vi "CRYPIC CLOSE SPLITER.vi"(10 "tSpliter":T1) -> (2 "tSpliter_Out":T1)   [LabVIEW 2013]
uses:
  CRYMain Sub Window Global.vi
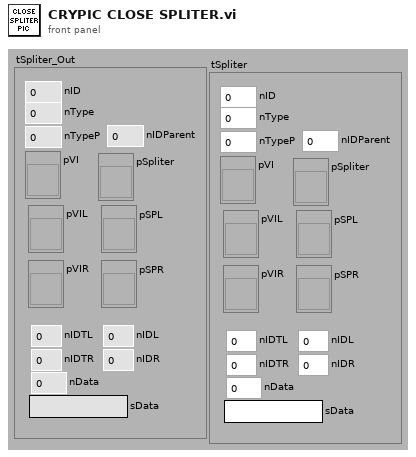
[diagram p1: front panel]
types:
  T1 = cluster{"nType":i32, "nTypeP":i32, "pVI":refnum<vi>, "pSpliter":refnum<vi>, "pSPL":refnum<vi>, "pVIL":refnum<vi>, "pSPR":refnum<vi>, "pVIR":refnum<vi>, "nIDTL":i32, "nIDL":i32, "nIDTR":i32, "nIDR":i32, "nID":i32, "nIDParent":i32, "nData":i32, "sData":string}
  T2 = cluster{"nID":i32[], "Spliter":cluster{"nType":i32, "nTypeP":i32, "pVI":refnum<vi>, "pSpliter":refnum<vi>, "pSPL":refnum<vi>, "pVIL":refnum<vi>, "pSPR":refnum<vi>, "pVIR":refnum<vi>, "nIDTL":i32, "nIDL":i32, "nIDTR":i32, "nIDR":i32, "nID":i32, "nIDParent":i32, "nData":i32, "sData":string}[]}
  T3 = cluster{"nType":i32, "nTypeP":i32, "pVI":refnum<vi>, "pSpliter":refnum<vi>, "pSPL":refnum<vi>, "pVIL":refnum<vi>, "pSPR":refnum<vi>, "pVIR":refnum<vi>, "nIDTL":i32, "nIDL":i32, "nIDTR":i32, "nIDR":i32, "nID":i32, "nIDParent":i32, "nData":i32, "sData":string}[]
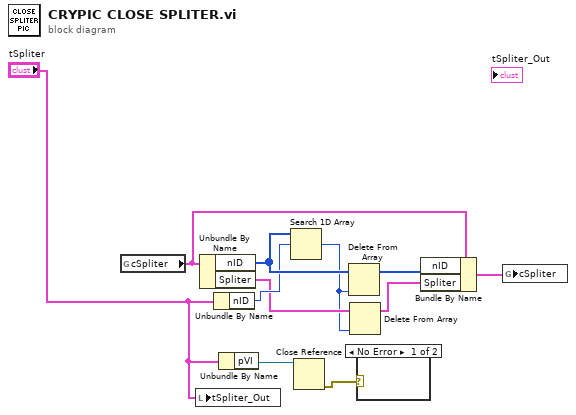
[diagram p0: block diagram]
diagram:
  n1 = global read "CRYMain Sub Window Global.vi" "cSpliter"() -> (w10:T2)
  n2 = local write "tSpliter_Out"("tSpliter") -> ()
  n3 = Unbundle By Name(w10) -> ("nID"=w9:i32[], "Spliter"=w6:T3)
  n4 = Unbundle By Name("tSpliter") -> ("nID"=w8:i32)
  n5 = Unbundle By Name("tSpliter") -> ("pVI"=w2:refnum<vi>)
  n6 = Search 1D Array(1D array=w9, element=w8) -> (index of element=w5:i32)  [unwired: 1 out]
  n7 = Close Reference(reference=w2) -> (error out=w1:errorcluster)  [unwired: 1 in]
  n8 = Delete From Array(array=w9, index=w5) -> (array with subset deleted=w11:i32[])  [unwired: 1 in, 1 out]
  n9 = Delete From Array(array=w6, index=w5) -> (array with subset deleted=w7:T3)  [unwired: 1 in, 1 out]
  n10 = case shown="No Error" w1 {
    frame No Error {
    }
    frame Error {
    }
  }
  n11 = Bundle By Name(cluster=w10, "nID"=w11, "Spliter"=w7) -> (w4:T2)
  n12 = global write "CRYMain Sub Window Global.vi" "cSpliter"(w4) -> ()
